vi "grabber.vi"() -> ()   [LabVIEW 2010]
uses:
  config_data_cluster.ctl
  <vilib>/Platform/TimedLoop/XDataNode/XDataNode.xnode
  <vilib>/Platform/TimedLoop/XDataNode/timing_clust.ctl
  <vilib>/Platform/TimedLoop/XDataNode/nitl_modes.ctl
  <vilib>/Platform/TimedLoop/XDataNode/wakeup.ctl
  <vilib>/dex/Flush And Wait Empty Condition.ctl
  <vilib>/rvi/interface/nirviMethod/nirviMethod.xnode
  <vilib>/rvi/interface/nirviReadWriteControl/nirviReadWriteControl.xnode
  <vilib>/rvi/interface/common/niFpgaNodeNameForErrorReporting.ctl
  <vilib>/rvi/errors/niLvFpgaWhatHappensToTopLevelVI.ctl
  <vilib>/rvi/interface/nirviCloseFPGA/nirviCloseFPGA.xnode
  <vilib>/Utility/error.llb/Error Cluster From Error Code.vi
  <vilib>/rvi/errors/niLvFpgaAdjustHostInterfaceError.vi
  <vilib>/FPGAPlugInAG/Dynamic/niLvFpga_Close_Dynamic.vi
  <vilib>/Platform/TimedLoop/XDataNode/XDNodeRunTimeDep.lvlib
  NiFpgaLv.dll
panel:
  in  "Mark fly-forward phase?":bool
  in  "adjust N sums":u32=100 max=10000 step=20
  in  "fake image fast loop?":bool
  out "ch0":u16[](graph)
  in  "Transpose graph view?":bool
  in  "Display green and red PMT?":bool
  in  "pick last TAG slice":u32
  in  "pick first TAG slice":u32
  in  "choose TAG slice?":bool
  in  "set ch1 max value":dbl
  in  "set ch0 max value":dbl
  out "ch1:position X":dbl
  out "ch0:position X":dbl
  in  "Adjust TAG phase":bool
  out "TAG profile at position X":dbl[][](graph)
  out "channel1":dbl[][](graph)
  out "channel0":dbl[][](graph)
  in  "N sums":u32(slide)=100 scale=0.0..100.0
  out "loop time":u32
  out "y galvo":i16(graph)
  out "scan specification":T1={"x amplitude"=100, "x resolution (pixels)"=28, "x offset fly-forward (iterations)"=50, "x offset fly-back (iterations)"=100, "y resolution (nr. of lines)"=80, "y step size"=30, "iterations per pixel"=5, "number of frames"=-1, "y offset (pixels)"=0, "number of y-brake lines  (before y-fly-back)"=0, "number y-brake lines (after y-fly-back)"=40, "number of y-fly-back steps"=0, "lines per z step"=1, "number of z/intensity tuples"=228, "number of repetitions (volumes or planes)"=-1, "z step size derived"=32, "choose the beginning of z scan"=FALSE, "number of frames (settings)"=80, "FPGA trajectory?"=TRUE, "Pockels cell voltage (bits)"=0, "Vy min(bits)"=0, "Vz min(bits)"=0}
  out "channel data block 2":dbl[][](graph)
  in  "fake image?":bool
  in  "xy view?":bool
  in  "Pockels cell voltage":i16(slide) min=-750 max=750 step=5 scale=-750.0..750.0
  out "DAC voltages":T2
  out "no. of extra wait lines written to FPGA FIFO":i32
  out "no. of z/int tuples written to FPGA FIFO":i32
  out "number of update commands received":i32
  out "extra wait lines set":bool
  out "zIntensity tuples set":bool
  out "scan spec set":bool
  out "display loop finished":bool
  in  "stop acquisition at FIFO overflow?  GRABBER":bool
  out "acquire?":bool
  out "FIFO overflow":bool
  out "scan":bool
  out "stop FPGA":bool
  out "wait for trigger?":bool
  out "stop acquisition at FIFO overflow?":bool
  out "scanning? FPGA":bool
  out "counter cluster out":T3
  out "extra waitlines array entries":u32[](graph)
  out "extra waitlines received by FPGA":u32
  out "no. of extra waitlines received":i32
  out "no of correctly transferred z tuples":u32
  out "z-points transfer corrupt?":bool
  out "intensity values":u16[](graph)
  out "z values":u16[](graph)
  out "no. of z/int. tubles received":i32
  out "z/intensity tuples received by FPGA":u32
  in  "wait till update":u32=500
  out "configuration":T4
  out "read FIFO overflow duration [ms]":u32
  out "read pixels duration [ms]":u32
  out "stream pixels [ms]":u32
  in  "Close front-panel?":bool=TRUE
  out "initialised?":bool
  in  "stop":bool
  out "command lp err":errorcluster
  out "error out":errorcluster
  out "effective read-block size":u32
  in  "max read block size":u32=32000
  out "read loop ctr":i32
  out "pixels read from FPGA":u64
  out "elements in FPGA FIFO":u32
  out "last received command":string
  out "command loop finished":bool
  out "read loop finished":bool
  out "scanning?":bool
  out "FIFO overflow?":bool
  out "data read from FPGA FIFO":u32[](array[numeric])
  # "enter a number between -+750V"
  # "Sum a single frame N times before displaying:"
  # "ms"
  # "automatically sets N=100 sums, otherwise FPGA buffer overflow"
  # "When T: displays and saves ch0.bin= green and ch1.bin =red\nWhen F: displays and saves ch0.bin= greenFF  and ch1.bin= greenFB  (FF=fly-forward and FB=fly-back)"
  # "Use when you want to display and save green and red PMT with marked FF and FB phases\nWhen T: fly-forward=photon counts+2^15 (number 1 at U16's most significant value)\n               and fly-back=photon counts\nWhen F: saves true photon count in both FF and FB phases of the red and green channel"
  # "How to use:\nTo adjust TAG phase\n1. set \"xy gavlo view?\"=F\n2. adjust Tag phase? = T\n3. drag cursor to desired x position\n   -- indicator below\n4. check z profile on the graph\n5. when done set N=0"
  # "How to use:\n1. set \"xy gavlo view?\"=T\n    on the main HS window\n2. to display xy view, sum all z stacks\n          set xy view?=T\n3. to choose a range of z slices to sum\na) xy view?=T\nb)choose TAG slice?=T\nc)eg. pick first Tag slice=3, pick last TAG slice=5\n   -> sums 3+4+5\nd) to display just one slice \n     set \"first=last\""
  # "RealTime Grabber"
  # "Status"
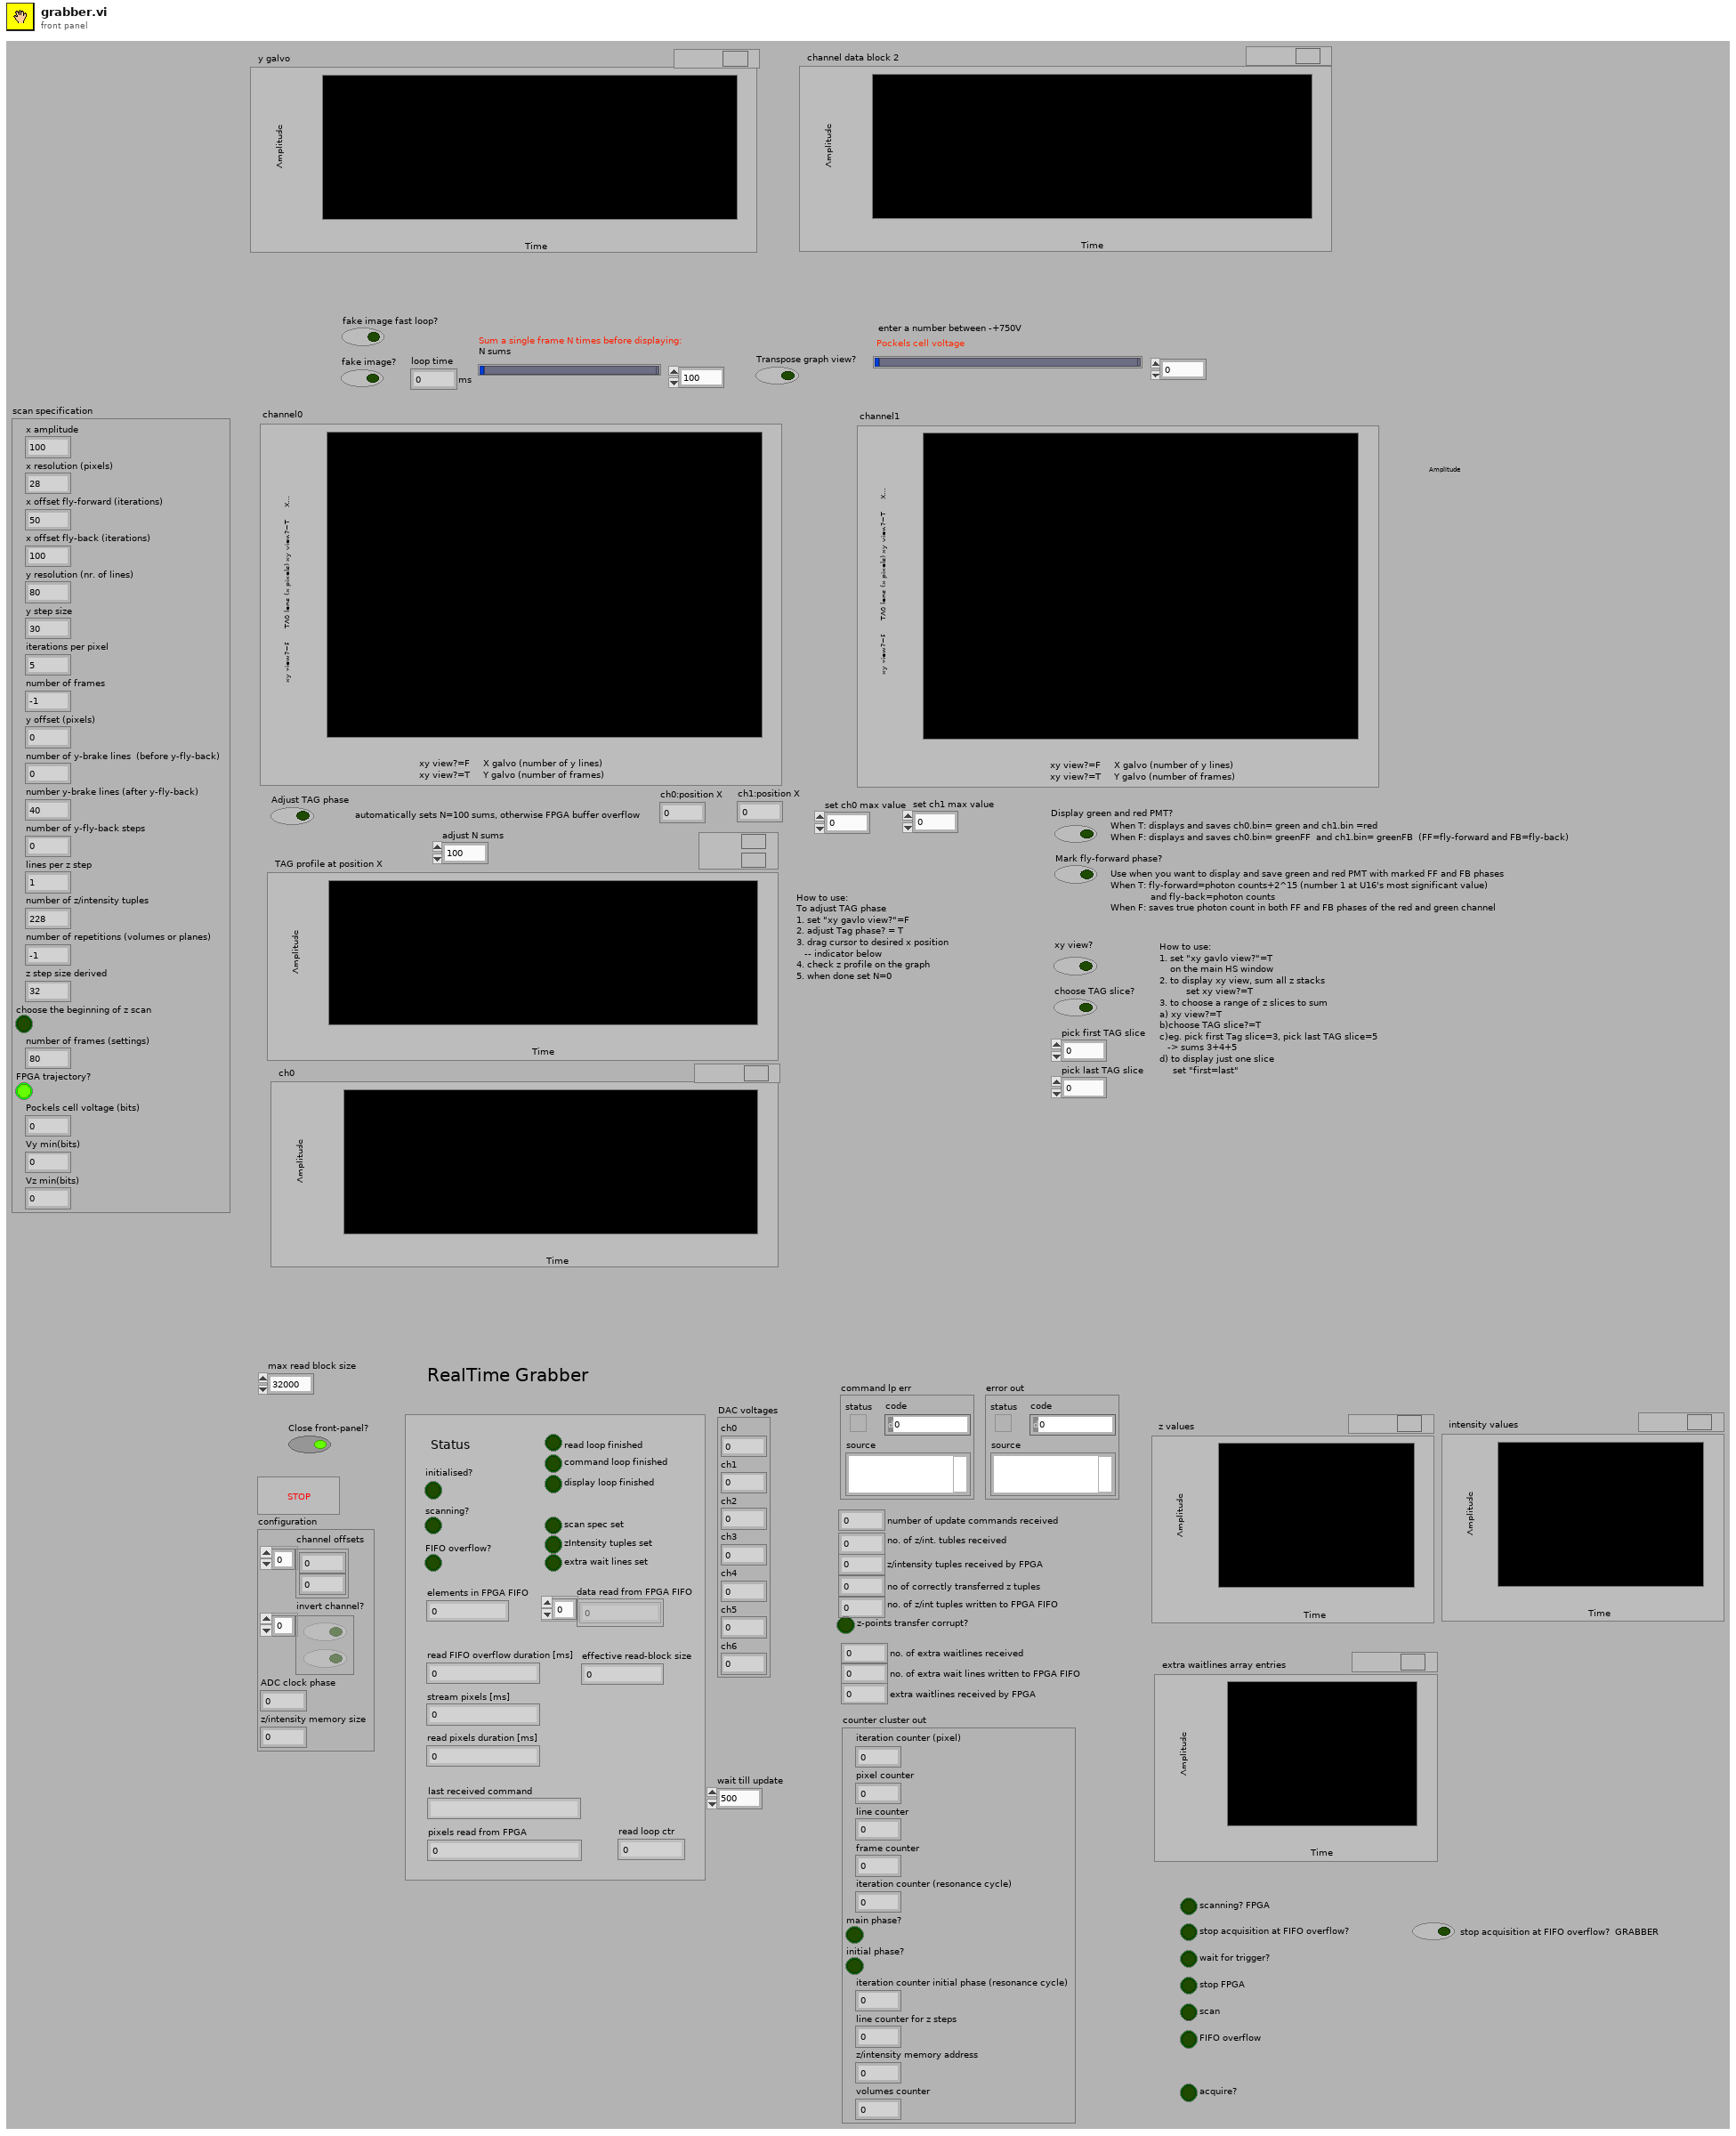
[diagram p1: front panel]
types:
  T1 = cluster{"x amplitude":u16, "x resolution (pixels)":u16, "x offset fly-forward (iterations)":u16, "x offset fly-back (iterations)":u16, "y resolution (nr. of lines)":u16, "y step size":u16, "iterations per pixel":u16, "number of frames":i32, "y offset (pixels)":u16, "number of y-brake lines  (before y-fly-back)":u16, "number y-brake lines (after y-fly-back)":u16, "number of y-fly-back steps":u16, "lines per z step":u16, "number of z/intensity tuples":u16, "number of repetitions (volumes or planes)":i32, "z step size derived":u16, "choose the beginning of z scan":bool, "number of frames (settings)":i32, "FPGA trajectory?":bool, "Pockels cell voltage (bits)":i16, "Vy min(bits)":i16, "Vz min(bits)":i16}
  T2 = cluster{"ch0":u16, "ch1":i16, "ch2":i16, "ch3":i16, "ch4":u16, "ch5":u16, "ch6":u16}
  T3 = cluster{"iteration counter (pixel)":u16, "pixel counter":u16, "line counter":u16, "frame counter":u16, "iteration counter (resonance cycle)":u16, "main phase?":bool, "initial phase?":bool, "iteration counter initial phase (resonance cycle)":u16, "line counter for z steps":u16, "z/intensity memory address":u32, "volumes counter":u16}
  T4 = typedef "config_data_cluster.ctl" = cluster{"channel offsets":u32[], "invert channel?":bool[], "ADC clock phase":i32, "z/intensity memory size":i32}
  T5 = typedef "network_streaming_queues_cluster.ctl" = cluster{"data writer endpoint":refnum<k21>, "command reader endpoint":refnum<k21>, "settings reader endpoint":refnum<k21>, "z/intensity tuples reader endpoint":refnum<k21>, "extra waitlines reader endpoint":refnum<k21>}
  T6 = typedef "XDNodeRunTimeDep.lvlib/timing_clust.ctl" = cluster{"Expected End [f-1]":u64, "Actual End [f-1]":u64, "Finished Late? [f-1]":bool, "Expected End [i-1]":u64, "Actual End [i-1]":u64, "Finished Late? [i-1]":bool, "Expected Start [i]":u64, "Actual Start [i]":u64, "Expected Start [f]":u64, "Actual Start [f]":u64, "Source Name":string, "Structure Name":string, "Period":i64, "Deadline":i64, "Offset":i64, "Start":i64, "Priority":i32, "Timeout":i32, "Mode":T7, "Wakeup Reason":T8, "Error":errorcluster, "Source Type":string, "Secondary Source Type":string, "Global End Time":u64, "Global Start Time":u64, "Frame Duration":u64, "Iteration Duration":u64, "Assigned CPU":i32, "I/O Scan Engine Mode":u32}
  T7 = typedef "XDNodeRunTimeDep.lvlib/nitl_modes.ctl" = enum32{"No Change", "Process missed periods, maintain original phase", "Discard missed periods, maintain original phase", "Process missed periods, ignore original phase", "Discard missed periods, ignore original phase"}
  T8 = typedef "XDNodeRunTimeDep.lvlib/wakeup.ctl" = enum32{"Normal", "Aborted", "Asynchronous wakeup", "Timing source error", "Timed loop error", "Timeout"}
  T9 = typedef "niFpgaNodeNameForErrorReporting.ctl" = enum16{"Open FPGA VI Reference", "Read/Write Control", "Invoke Method: Abort", "Invoke Method: Acknowledge IRQ", "Invoke Method: Download", "Invoke Method: FIFO.Configure", "Invoke Method: FIFO.Read", "Invoke Method: FIFO.Start", "Invoke Method: FIFO.Stop", "Invoke Method: FIFO.Write", "Invoke Method: Reset", "Invoke Method: Run", "Invoke Method: Wait on IRQ", "Close FPGA VI Reference"}
  T10 = typedef "niLvFpgaWhatHappensToTopLevelVI.ctl" = enum16{"top level VI scripted behind XNode", "top level VI inlined behind XNode"}
  T11 = typedef "Flush And Wait Empty Condition.ctl" = u8
  T12 = typedef "scan_specification_cluster.ctl" = cluster{"x amplitude":u16, "x resolution (pixels)":u16, "x offset fly-forward (iterations)":u16, "x offset fly-back (iterations)":u16, "y resolution (nr. of lines)":u16, "y step size":u16, "iterations per pixel":u16, "number of frames":i32, "y offset (pixels)":u16, "number of y-brake lines  (before y-fly-back)":u16, "number y-brake lines (after y-fly-back)":u16, "number of y-fly-back steps":u16, "lines per z step":u16, "number of z/intensity tuples":u16, "number of repetitions (volumes or planes)":i32, "z step size derived":u16, "choose the beginning of z scan":bool, "number of frames (settings)":i32, "FPGA trajectory?":bool, "Pockels cell voltage (bits)":i16, "Vy min(bits)":i16, "Vz min(bits)":i16}
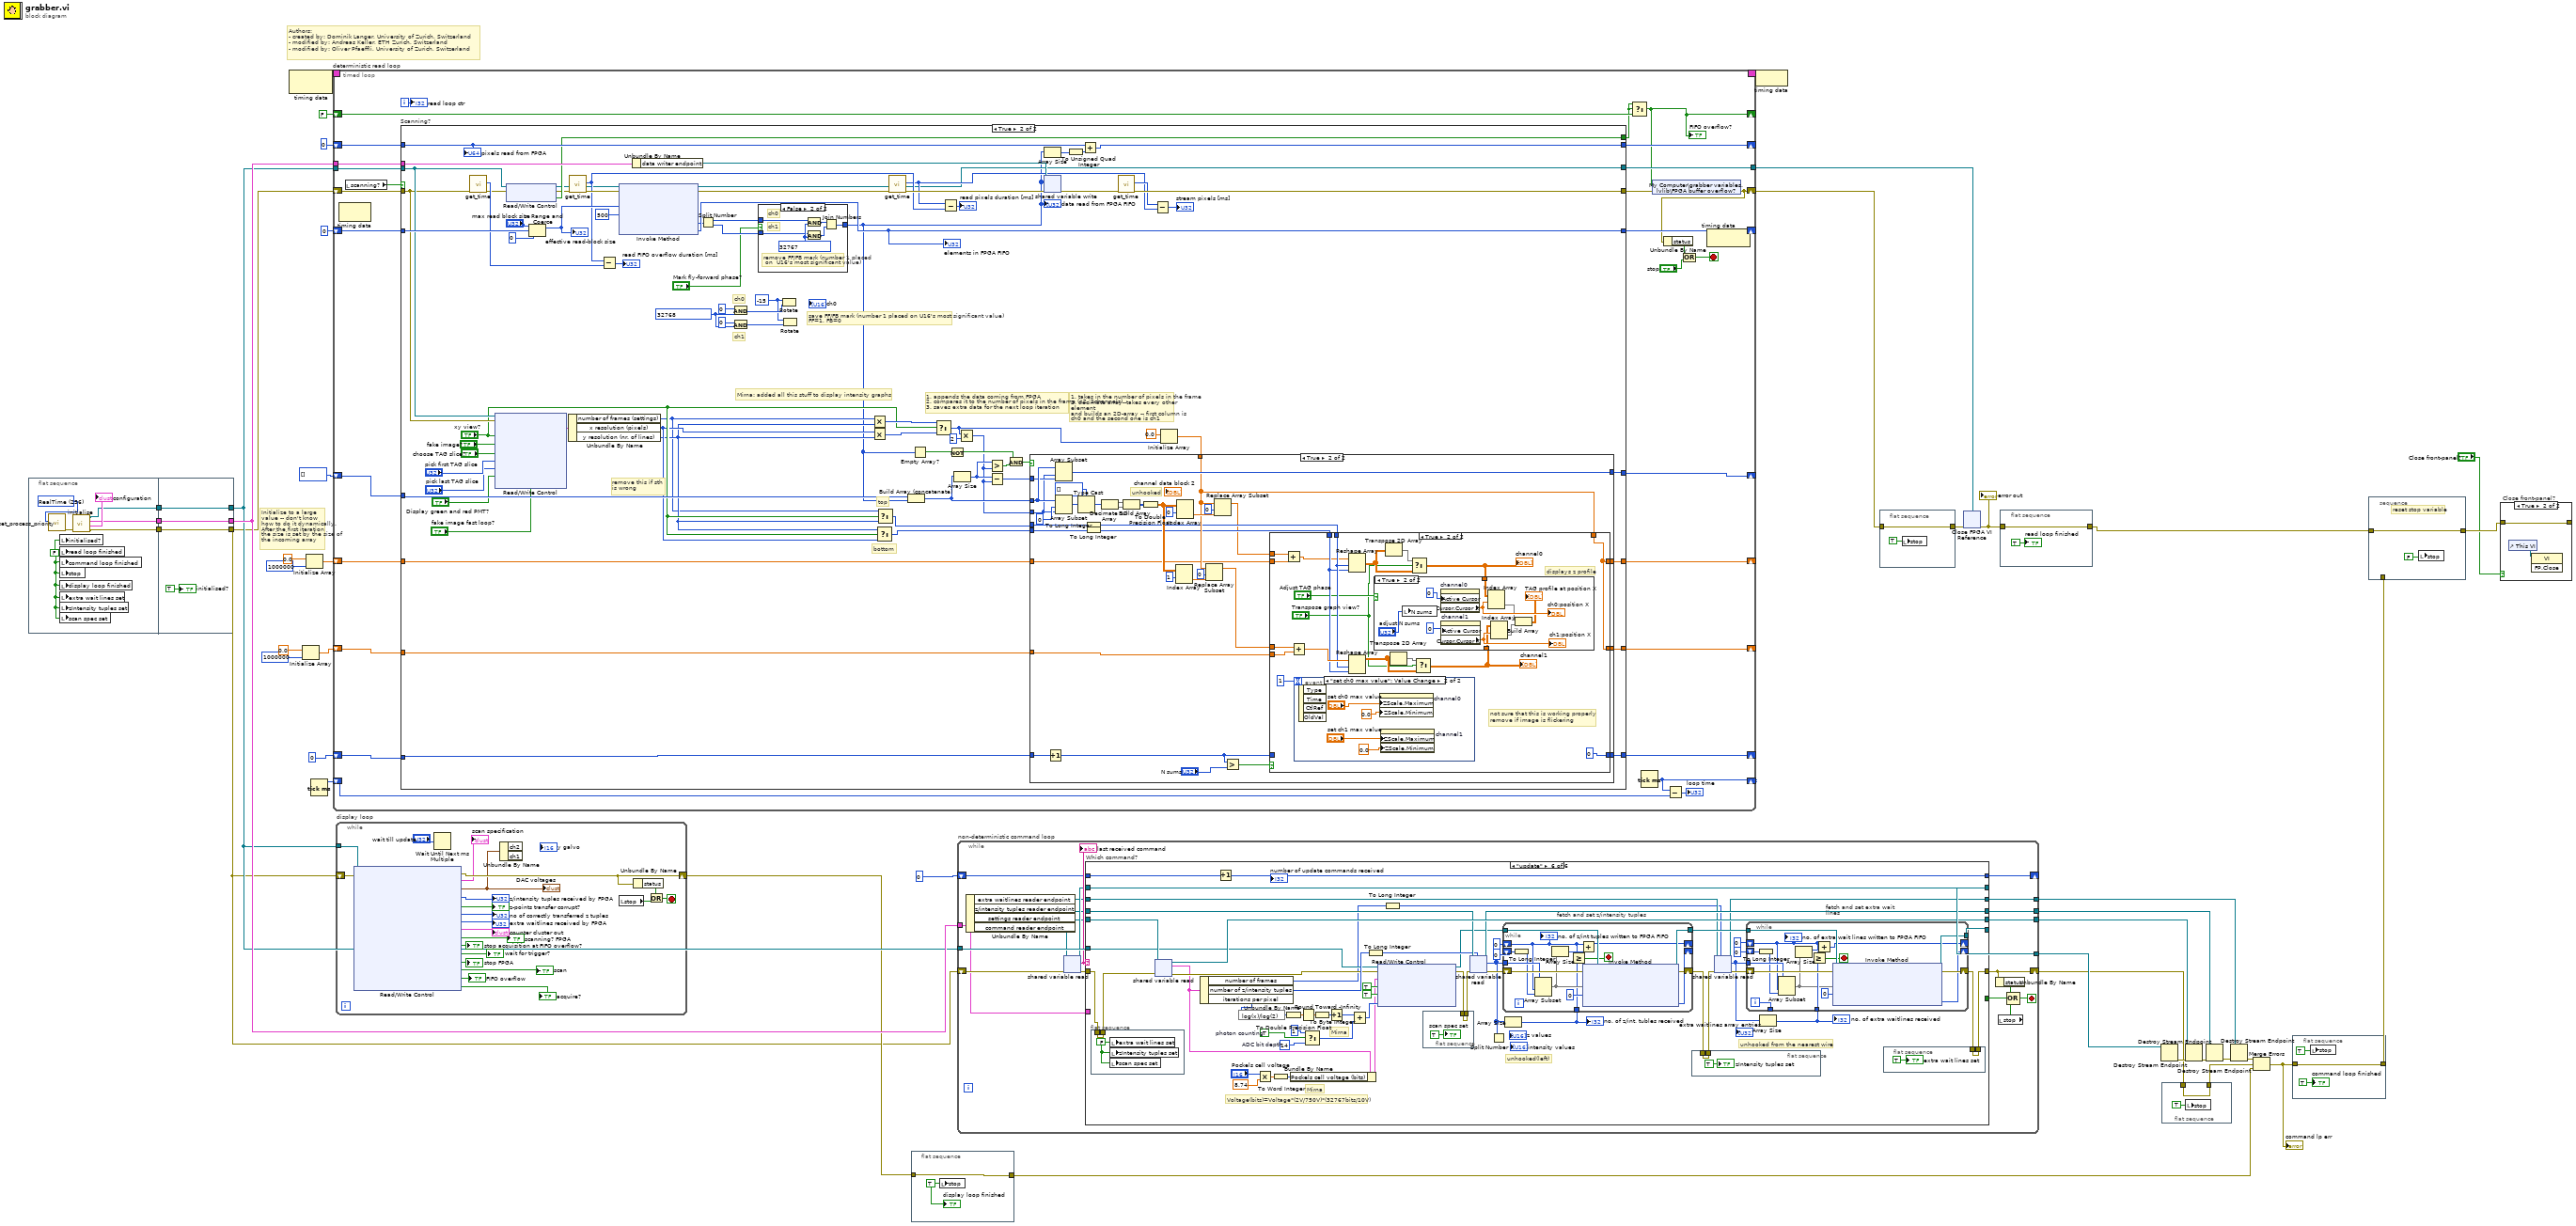
[diagram p0: block diagram]
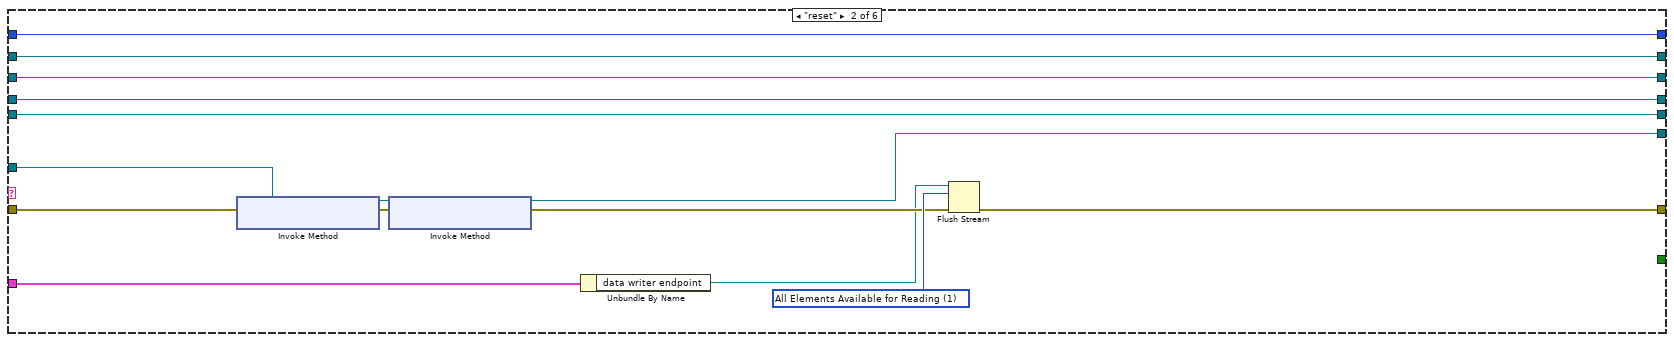
[diagram p4: hidden frame]
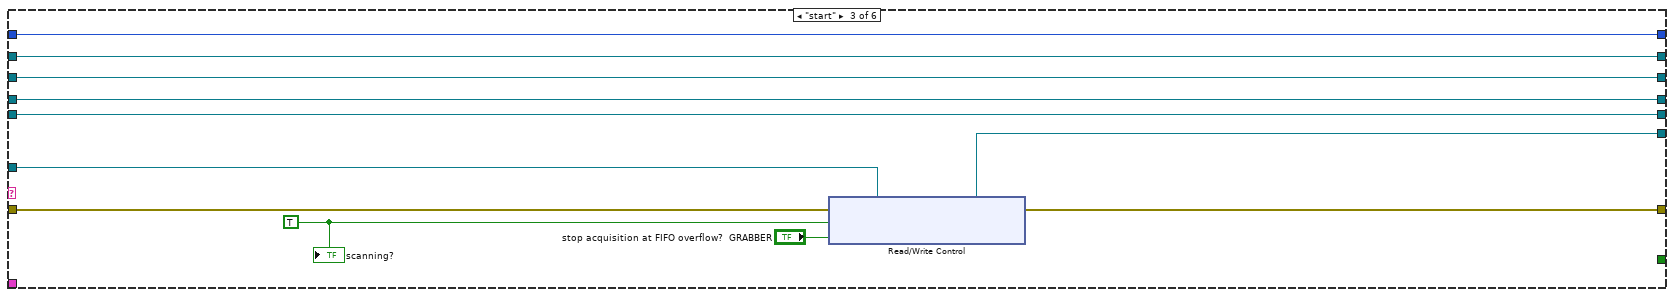
[diagram p5: hidden frame]
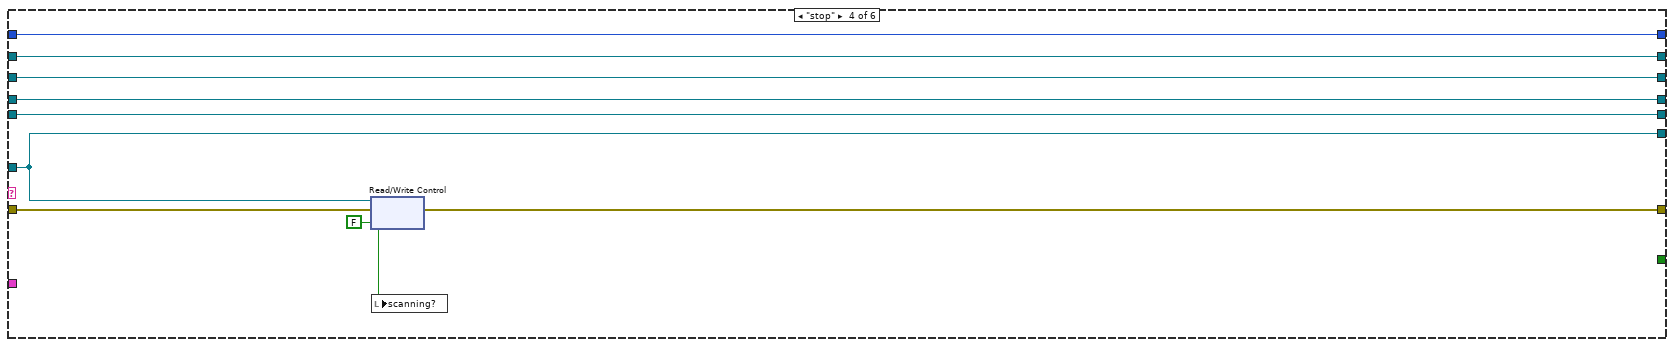
[diagram p6: hidden frame]
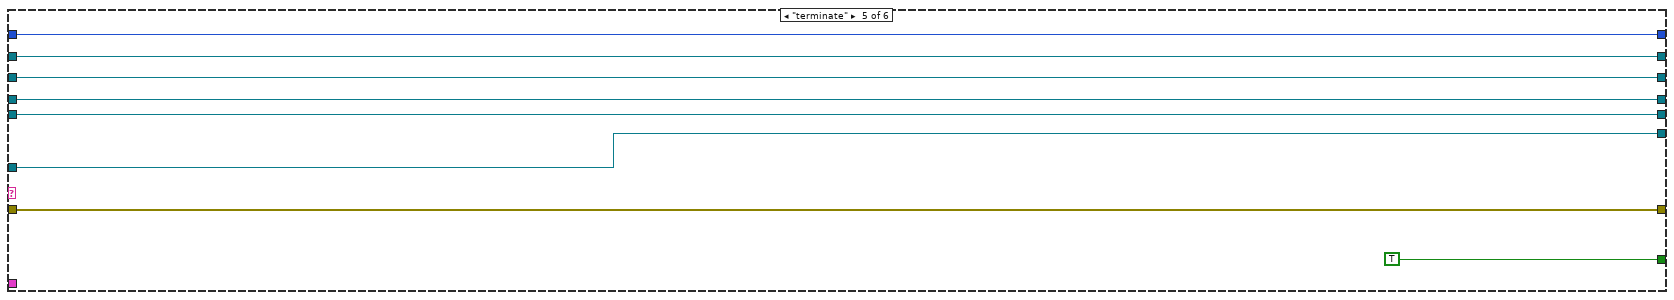
[diagram p7: hidden frame]
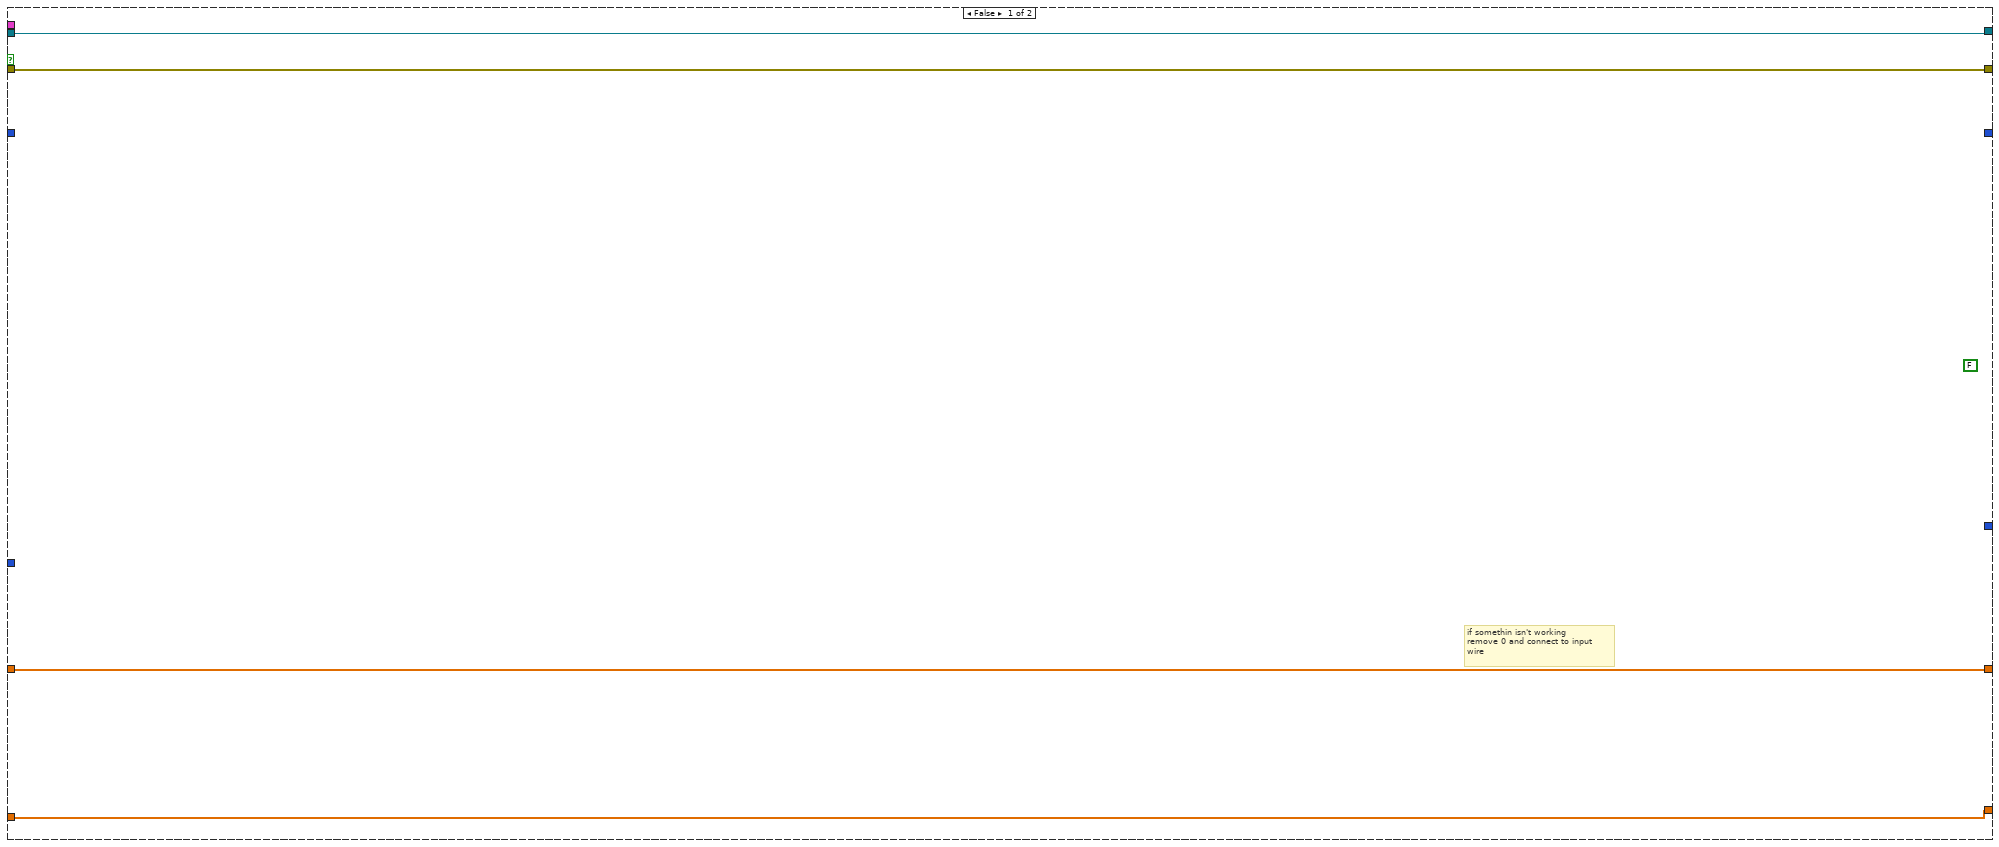
[diagram p8: hidden frame]
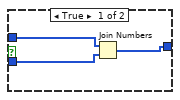
[diagram p9: hidden frame]
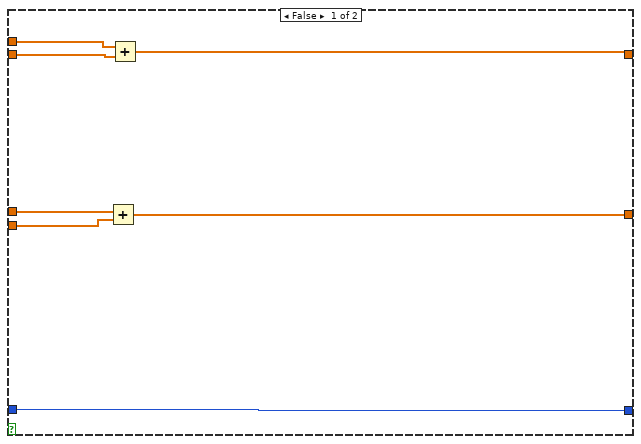
[diagram p11: hidden frame]
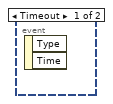
[diagram p12: hidden frame]
diagram:
  # "Initialize to a large \nvalue -- don't know \nhow to do it dynamically.\nAfter the first iteration\nthe size is set by the size of\nthe incoming array"
  # "Authors: \n- created by: Dominik Langer, University of Zurich, Switzerland\n- modified by: Andreas Keller, ETH Zurich, Switzerland\n- modified by: Oliver Pfaeffli, University of Zurich, Switzerland"
  n1 = flat-sequence {
    tunnel: [w47] -> w33
    tunnel: [w44] -> w32
    tunnel: [w45] -> w29
    tunnel: [w52] -> w22
    tunnel: [w53] -> w1
    tunnel: w33 -> [w53]
    tunnel: w32 -> [w52]
    tunnel: [w50] -> w28
    tunnel: w29 -> [w50]
    frame #0 {
      w43 = FALSE ("read loop finished")
      w49 = 256 items=["Normal"=32, "Idle"=64, "High"=128, "RealTime"=256, "BelowNormal"=16384, "AboveNormal"=32768] ("PriorityClass")
      n2 = call "set_process_priority.vi"("PriorityClass"=w49) -> ("error out"=w48:errorcluster)  [unwired: 10 in]
      n3 = local write "initialised?"(w43) -> ()
      n4 = local write "read loop finished"(w43) -> ()
      n5 = local write "command loop finished"(w43) -> ()
      n6 = local write "stop"(w43) -> ()
      n7 = local write "display loop finished"(w43) -> ()
      n8 = local write "extra wait lines set"(w43) -> ()
      n9 = local write "zIntensity tuples set"(w43) -> ()
      n10 = local write "scan spec set"(w43) -> ()
      n11 = call "initialise.vi"("error in (no error)"=w48) -> ("error out"=w47:errorcluster, "configuration"=→"configuration":T4, "network streaming queues"=w45:T5, "FPGA VI Reference Out"=w44:refnum<k20>)  [unwired: 6 in]
    }
    frame #1 {
      "initialised?" <- TRUE ("initialised?")
    }
  }
  n12 = node-c288 ("Input Node")() -> (w42:T6)  [unwired: 1 in]
  n13 = Initialize Array(0.0 ("element"), 1000000 ("dimension size")) -> (w9:dbl[])
  n14 = Initialize Array(0.0 ("element"), 1000000 ("dimension size")) -> (w3:dbl[])
  n15 = Tick Count (ms)() -> (millisecond timer value=w6:u32)
  n16 = timed-loop "deterministic read loop" {
    timing: w42 -> [_]
    timing-out: [_] -> w41
    shift-right: [w69] -> w21
    shift-left: w1 -> [w75]
    tunnel: w22 -> [w70]
    shift-right: [w56] -> _
    shift-left: FALSE ("FIFO overflow") -> [w82]
    shift-right: [w79] -> _
    shift-left: u64 0 -> [w81]
    tunnel: [w77] -> w35
    shift-right: [w73] -> _
    shift-left: u32 0 ("Elements Remaining") -> [w72]
    tunnel: w28 -> [w71]
    shift-right: [w64] -> _
    shift-left: u32[] [] -> [w65]
    shift-right: [w63] -> _
    shift-left: w9 -> [w62]
    shift-right: [w60] -> _
    shift-left: u32 0 ("Elements Remaining") -> [w61]
    shift-right: [w59] -> _
    shift-left: w6 -> [w58]
    shift-right: [w54] -> _
    shift-left: w3 -> [w55]
    i -> [w80]
    stop <- w66 stop-if-true
    n17 = node-c288 ("Output Node")() -> ()  [unwired: 1 in, 1 out]
    n18 = local read "scanning?"() -> (w74:bool)
    n19 = case "Scanning?" shown="True" w74 {
      tunnel: w75 -> [w88 w121]
      tunnel: [w88 w149] -> w76
      tunnel: w70 -> [w87 w135]
      tunnel: [w87 w137] -> w77
      tunnel: w81 -> [_ w157]
      tunnel: [_ w164] -> w79
      tunnel: [_ w140] -> w78
      tunnel: [_ w159] -> w73
      tunnel: w72 -> [_ w158]
      tunnel: w71 -> [_ w155]
      tunnel: w65 -> [_ w124]
      tunnel: [_ w123] -> w64
      tunnel: w62 -> [w85 w116]
      tunnel: [w85 w117] -> w63
      tunnel: w61 -> [_ w113]
      tunnel: [_ w115] -> w60
      tunnel: w55 -> [w86 w112]
      tunnel: [w86 w111] -> w54
      frame False {
        (unwired) FALSE ("FIFO overflow")
        # "if somethin isn't working \nremove 0 and connect to input \nwire"
      }
      frame True {
        w93 = i8 -15 ("y")
        w97 = u16 32768
        # "save FF/FB mark (number 1 placed on U16's most significant value)\nFF=1, FB=0"
        # "ch1"
        # "ch0"
        # "top"
        # "bottom"
        # "remove this if sth \nis wrong"
        # "1. takes in the number of pixels in the frame\n2. decimate array--takes every other element\nand builds an 2D-array -- first column is \nch0 and the second one is ch1"
        # "1. appends the data coming from FPGA\n2. compares it to the number of pixels in the frame (x2, 2channels)\n3. saves extra data for the next loop iteration"
        # "Mirna: added all this stuff to display intensity graphs"
        n20 = call "get_time.vi"("error in (no error)"=w121) -> ("error out"=w141:errorcluster, "millisecond timer value"=w145:u32)  [unwired: 9 in]
        n21 = xnode "Read/Write Control"("FPGA VI Reference In"=w135, "error in"=w121, "xy view?"="xy view?", "fake image?"="fake image?", "choose TAG slice?"="choose TAG slice?", "pick first TAG slice"="pick first TAG slice", "pick last TAG slice"="pick last TAG slice", "ch0-ch1?"="Display green and red PMT?", "fake image fast loop?"="fake image fast loop?") -> ("scan specification"=w136:T1)  [unwired: 2 out]
        n22 = xnode "Read/Write Control"("FPGA VI Reference In"=w135, "error in"=w141) -> ("FPGA VI Reference Out"=w138:refnum<k20>, "error out"=w139:errorcluster, "FIFO overflow"=w140:bool)
        n23 = In Range and Coerce(upper limit="max read block size", x=w158, lower limit=u32 0) -> (coerced(x)=w156:u32)  [unwired: 1 out]
        "effective read-block size" <- w156
        n24 = Unbundle By Name(w136) -> ("number of frames (settings)"=w101:i32, "x resolution (pixels)"=w104:u16, "y resolution (nr. of lines)"=w102:u16)
        n25 = call "get_time.vi"("error in (no error)"=w139) -> ("error out"=w147:errorcluster, "millisecond timer value"=w143:u32)  [unwired: 9 in]
        n26 = Subtract(x=w143, y=w145) -> (x-y=→"read FIFO overflow duration [ms]":u32)
        n27 = xnode "Invoke Method"("FPGA VI Reference In"=w138, "error in"=w147, "Number of Elements"=w156, "Timeout (ms)"=500) -> ("FPGA VI Reference Out"=w137:refnum<k20>, "error out"=w152:errorcluster, "Data"=w100:u32[], "Elements Remaining"=w159:u32)
        "elements in FPGA FIFO" <- w159
        n28 = Unbundle By Name(w155) -> ("data writer endpoint"=w154:refnum<k21>)
        n29 = Split Number(x=w100) -> (hi(x)=w98:u16[], lo(x)=w96:u16[])
        n30 = And(x=u16 0, y=w97) -> (x .and. y?=w95:u16)
        n31 = And(x=u16 0, y=w97) -> (x .and. y?=w94:u16)
        n32 = case shown="False" "Mark fly-forward phase?" {
          tunnel: [w166 w172] -> w99
          tunnel: w98 -> [w168 w170]
          tunnel: w96 -> [w167 w169]
          frame True {
            n33 = Join Numbers(hi=w168, lo=w167) -> ((hi.lo)=w166:u32[])
          }
          frame False {
            w174 = u16 32767
            # "ch1"
            # "ch0"
            # "remove FF/FB mark (number 1 placed\n on  U16's most significant value)"
            n34 = And(x=w170, y=w174) -> (x .and. y?=w173:u16[])
            n35 = And(x=w169, y=w174) -> (x .and. y?=w171:u16[])
            n36 = Join Numbers(hi=w173, lo=w171) -> ((hi.lo)=w172:u32[])
          }
        }
        "data read from FPGA FIFO" <- w99
        n37 = Rotate(1:w95, 2:w93) -> ()  [unwired: 1 out]
        n38 = Rotate(1:w94, 2:w93) -> ()  [unwired: 1 out]
        n39 = Multiply(x=w101, y=w102) -> (x*y=w119:i32)
        n40 = Multiply(x=w104, y=w102) -> (x*y=w128:u16)
        n41 = Select(t=w102, s="xy view?", f=w104) -> (s? t:f=w105:u16)
        n42 = Select(t=w101, s="xy view?", f=w102) -> (s? t:f=w103:i32)
        n43 = call "get_time.vi"("error in (no error)"=w152) -> ("error out"=w151:errorcluster, "millisecond timer value"=w142:u32)  [unwired: 9 in]
        n44 = Build Array (concatenate)(w124, w99) -> (w129:u32[])
        n45 = Empty Array?(array=w99) -> (empty?=w133:bool)
        n46 = Select(t=w119, s="xy view?", f=w128) -> (s? t:f=w120:i32)
        n47 = Subtract(x=w142, y=w143) -> (x-y=→"read pixels duration [ms]":u32)
        n48 = Not(x=w133) -> (.not. x?=w130:bool)
        n49 = Array Size(array=w129) -> (size(s)=w132:i32)
        n50 = Multiply(x=w120, y=u16 2) -> (x*y=w125:i32)
        n51 = Greater?(x=w132, y=w125) -> (0:w131:bool)
        n52 = Subtract(x=w132, y=w125) -> (x-y=w126:i32)
        n53 = And(x=w130, y=w131) -> (x .and. y?=w114:bool)
        n54 = shared-variable-write(w154, w151, w99) -> (w150:errorcluster)  [unwired: 1 in, 2 out]
        n55 = Array Size(array=w99) -> (size(s)=w165:i32)
        n56 = To Unsigned Quad Integer(1:w165) -> (0:w163:u64)
        n57 = Add(x=w157, y=w163) -> (x+y=w164:u64)
        n58 = call "get_time.vi"("error in (no error)"=w150) -> ("error out"=w149:errorcluster, "millisecond timer value"=w148:u32)  [unwired: 9 in]
        n59 = Subtract(x=w148, y=w142) -> (x-y=→"stream pixels [ms]":u32)
        n60 = Initialize Array(0.0 ("element"), w120) -> (w118:dbl[])
        n61 = case shown="True" w114 {
          tunnel: w129 -> [w178 w211]
          tunnel: w125 -> [_ w209]
          tunnel: w126 -> [_ w210]
          tunnel: [w178 w208] -> w123
          tunnel: w103 -> [_ w202]
          tunnel: w105 -> [_ w201]
          tunnel: w118 -> [_ w187]
          tunnel: w116 -> [w177 w194]
          tunnel: [w177 w189] -> w117
          tunnel: [w176 w193] -> w115
          tunnel: w113 -> [w176 w192]
          tunnel: w112 -> [w175 w181]
          tunnel: [w175 w180] -> w111
          frame False {
          }
          frame True {
            # "unhooked"
            n62 = Increment(x=w192) -> (x+1=w179:u32)
            n63 = Array Subset(array=w211, index=w209, length=w210) -> (w208:u32[])
            n64 = Array Subset(array=w211, index=0, length=w209) -> (w196:u32[])
            n65 = Type Cast(type=u16[] [], x=w196) -> (*(type *) &x=w205:u16[])
            n66 = To Long Integer(number=w202) -> (32bit integer=w186:i32)
            n67 = To Long Integer(number=w201) -> (32bit integer=w185:i32)
            n68 = Decimate 1D Array(w205) -> (w207:u16[], w206:u16[])
            n69 = Build Array(w207, w206) -> (w204:u16[][])
            n70 = To Double Precision Float(number=w204) -> (double precision float=w200:dbl[][])
            n71 = Index Array(array=w200, index (row)=1 ("index (col)")) -> (element=w190:dbl[])  [unwired: 1 in]
            n72 = Index Array(array=w200, index (row)=0) -> (element=w198:dbl[])  [unwired: 1 in]
            n73 = Replace Array Subset(array=w187, new element=w190, index=0) -> (w183:dbl[])
            n74 = Replace Array Subset(array=w187, new element=w198, index=0) -> (w182:dbl[])
            n75 = Greater?(x=w179, y="N sums") -> (0:w188:bool)
            n76 = case shown="True" w188 {
              tunnel: w194 -> [w216 w238]
              tunnel: [w219 u32 0] -> w193
              tunnel: w183 -> [w218 w237]
              tunnel: [w217 w230] -> w189
              tunnel: w179 -> [w219 _]
              tunnel: w187 -> [_ w230]
              tunnel: w186 -> [_ w234]
              tunnel: w185 -> [_ w233]
              tunnel: w182 -> [w215 w232]
              tunnel: w181 -> [w214 w231]
              tunnel: [w213 w230] -> w180
              frame False {
                n77 = Add(x=w218, y=w216) -> (x+y=w217:dbl[])
                n78 = Add(x=w215, y=w214) -> (x+y=w213:dbl[])
              }
              frame True {
                # "displays z profile"
                # "not sure that this is working properly\nremove if image is flickering"
                n79 = Add(x=w232, y=w231) -> (x+y=w228:dbl[])
                n80 = Add(x=w237, y=w238) -> (x+y=w235:dbl[])
                n81 = event shown="[1] \"set ch0 max value\": Value Change" {
                  selector: _ -> [_ _]
                  dyn-events: _ -> [_ _]
                  timeout: 1 -> [_ _]
                  event Timeout {
                    n82 = event-data() -> ()  [unwired: 1 in, 2 out]
                  }
                  event "set ch0 max value": Value Change {
                    n83 = event-data() -> ()  [unwired: 1 in, 4 out]
                    n84 = property on="channel0" class="IntGraph (strict)"("ZScale.Maximum"="set ch0 max value", "ZScale.Minimum"=0.0 ("Z Scale.Range:Minimum")) -> ()  [unwired: 2 in, 2 out]
                    n85 = property on="channel1" class="IntGraph (strict)"("ZScale.Maximum"="set ch1 max value", "ZScale.Minimum"=0.0 ("Z Scale.Range:Minimum")) -> ()  [unwired: 2 in, 2 out]
                  }
                }
                n86 = Reshape Array(w228, w234, w233) -> (w224:dbl[][])
                n87 = Reshape Array(w235, w234, w233) -> (w221:dbl[][])
                n88 = Transpose 2D Array(2D array=w224) -> (transposed array=w226:dbl[][])
                n89 = Transpose 2D Array(2D array=w221) -> (transposed array=w223:dbl[][])
                n90 = Select(t=w226, s="Transpose graph view?", f=w224) -> (s? t:f=w225:dbl[][])
                "channel0" <- w225
                n91 = Select(t=w223, s="Transpose graph view?", f=w221) -> (s? t:f=w222:dbl[][])
                "channel1" <- w222
                n92 = case shown="True" "Adjust TAG phase" {
                  tunnel: w225 -> [_ w251]
                  tunnel: w222 -> [_ w245]
                  frame False {
                  }
                  frame True {
                    n93 = local write "N sums"("adjust N sums") -> ()
                    n94 = property on="channel0" class="IntGraph (strict)"("Active Cursor"=u32 0) -> ("Cursor.Cursor X"=w250:dbl)  [unwired: 2 in, 2 out]
                    "ch0:position X" <- w250
                    n95 = property on="channel1" class="IntGraph (strict)"("Active Cursor"=u32 0) -> ("Cursor.Cursor X"=w248:dbl)  [unwired: 2 in, 2 out]
                    "ch1:position X" <- w248
                    n96 = Index Array(array=w251, index (row)=w250) -> (element=w247:dbl[])  [unwired: 1 in]
                    n97 = Index Array(array=w245, index (row)=w248) -> (element=w246:dbl[])  [unwired: 1 in]
                    n98 = Build Array(w247, w246) -> (→"TAG profile at position X":dbl[][])
                  }
                }
              }
            }
          }
        }
        "pixels read from FPGA" <- w157
      }
    }
    n99 = Select(t=w78, s=w78, f=w82) -> (s? t:f=w56:bool)
    "FIFO overflow?" <- w56
    n100 = Tick Count (ms)() -> (millisecond timer value=w59:u32)
    n101 = shared-variable "My Computer\\grabber variables.lvlib\\FPGA buffer overflow?"(w56, error in=w76) -> (error out=w69:errorcluster)
    n102 = Unbundle By Name(w69) -> ("status"=w68:bool)
    n103 = Subtract(x=w59, y=w58) -> (x-y=→"loop time":u32)
    n104 = Compound Arithmetic op=OR(w68, "stop") -> (w66:bool)
    n105 = node-c288 ("Input Node")() -> ()  [unwired: 1 in, 1 out]
    "read loop ctr" <- w80
  }
  n106 = while "display loop" {
    tunnel: w22 -> [w591]
    shift-right: [w589] -> w19
    shift-left: w1 -> [w590]
    stop <- w586 stop-if-true
    n107 = xnode "Read/Write Control"("FPGA VI Reference In"=w591, "error in"=w590) -> ("error out"=w589:errorcluster, "scan specification"=→"scan specification":T1, "DAC voltages"=w572:T2, "transferred z/intensity tuples"=→"z/intensity tuples received by FPGA":u32, "z-points transfer corrupt?"=→"z-points transfer corrupt?":bool, "no of correct transferred z tuples"=→"no of correctly transferred z tuples":u32, "transferred extra waitlines"=→"extra waitlines received by FPGA":u32, "counter cluster out"=→"counter cluster out":T3, "scanning?"=→"scanning? FPGA":bool, "stop acquisition at FIFO overflow?"=→"stop acquisition at FIFO overflow?":bool, "wait for trigger?"=→"wait for trigger?":bool, "stop"=→"stop FPGA":bool, "scan"=→"scan":bool, "FIFO overflow"=→"FIFO overflow":bool, "acquire?"=→"acquire?":bool)  [unwired: 1 out]
    "DAC voltages" <- w572
    n108 = Wait Until Next ms Multiple(millisecond multiple="wait till update") -> ()  [unwired: 1 out]
    n109 = Unbundle By Name(w572) -> ()  [unwired: 2 out]
    n110 = local read "stop"() -> (w587:bool)
    n111 = Unbundle By Name(w589) -> ("status"=w588:bool)
    n112 = Or(x=w588, y=w587) -> (x .or. y?=w586:bool)
  }
  n113 = flat-sequence {
    tunnel: w19 -> [w983]
    tunnel: [w983] -> w18
    frame #0 {
      w982 = TRUE ("stop")
      n114 = local write "stop"(w982) -> ()
      "display loop finished" <- w982
    }
  }
  n115 = while "non-deterministic command loop" {
    shift-right: [w991] -> w17
    shift-left: w1 -> [w1004]
    tunnel: w22 -> [w1003]
    tunnel: [w999] -> w40
    tunnel: w28 -> [w997]
    tunnel: [w995] -> w25
    tunnel: [w993] -> w23
    tunnel: [w986] -> w13
    shift-right: [w984] -> _
    shift-left: 0 -> [w985]
    stop <- w989 stop-if-true
    n116 = Unbundle By Name(w997) -> ("extra waitlines reader endpoint"=w987:refnum<k21>, "z/intensity tuples reader endpoint"=w994:refnum<k21>, "settings reader endpoint"=w996:refnum<k21>, "command reader endpoint"=w998:refnum<k21>)
    n117 = shared-variable-read(w998, w1004) -> (w1000:refnum<k21>, w1002:errorcluster, w1001:string)  [unwired: 1 in, 1 out]
    "last received command" <- w1001
    n118 = case "Which command?" shown="\"update\"" w1001 {
      tunnel: w1003 -> [w1009 w1024 w1079 w1150 w1197 w1238]
      tunnel: w1002 -> [w1011 w1026 w1077 w1149 w1196 w1215]
      tunnel: [w1011 w1018 w1081 w1147 w1196 w1220] -> w991
      tunnel: w1000 -> [w1010 w1025 w1080 w1151 w1198 w1248]
      tunnel: [w1010 w1025 w1080 w1151 w1198 w1248] -> w999
      tunnel: [w1009 w1023 w1078 w1150 w1197 w1229] -> _
      tunnel: w997 -> [_ w1017 _ _ _ _]
      tunnel: w996 -> [w1008 w1015 w1075 w1146 w1195 w1247]
      tunnel: [w1008 w1015 w1075 w1146 w1195 w1246] -> w995
      tunnel: w994 -> [w1007 w1014 w1074 w1145 w1194 w1245]
      tunnel: [w1007 w1014 w1074 w1145 w1194 w1244] -> w993
      tunnel: [_ _ _ _ TRUE _] -> w992
      tunnel: w987 -> [w1006 w1013 w1073 w1144 w1192 w1227]
      tunnel: [w1006 w1013 w1073 w1144 w1192 w1226] -> w986
      tunnel: w985 -> [w1005 w1012 w1071 w1143 w1191 w1213]
      tunnel: [w1005 w1012 w1071 w1143 w1191 w1212] -> w984
      frame "NULL", Default {
      }
      frame "reset" {
        w1020 = T11 1 items=["All Elements Read From Stream", "All Elements Available for Reading"] ("wait condition")
        n119 = xnode "Invoke Method"("FPGA VI Reference In"=w1024, "error in"=w1026) -> ("FPGA VI Reference Out"=w1021:refnum<k20>, "error out"=w1022:errorcluster)
        n120 = xnode "Invoke Method"("FPGA VI Reference In"=w1021, "error in"=w1022) -> ("FPGA VI Reference Out"=w1023:refnum<k20>, "error out"=w1019:errorcluster)
        n121 = Unbundle By Name(w1017) -> ("data writer endpoint"=w1016:refnum<k21>)
        n122 = Flush Stream(8:w1019, 10:w1020, 11:w1016) -> (0:w1018:errorcluster)  [unwired: 1 in, 2 out]
      }
      frame "start" {
        w1076 = TRUE ("scan")
        n123 = xnode "Read/Write Control"("FPGA VI Reference In"=w1079, "error in"=w1077, "scan"=w1076, "stop acquisition at FIFO overflow?"="stop acquisition at FIFO overflow?  GRABBER") -> ("FPGA VI Reference Out"=w1078:refnum<k20>, "error out"=w1081:errorcluster)
        "scanning?" <- w1076
      }
      frame "stop" {
        w1148 = FALSE ("scan")
        n124 = xnode "Read/Write Control"("FPGA VI Reference In"=w1150, "error in"=w1149, "scan"=w1148) -> ("error out"=w1147:errorcluster)  [unwired: 1 out]
        n125 = local write "scanning?"(w1148) -> ()
      }
      frame "terminate" {
      }
      frame "update" {
        w1207 = TRUE  # photon counting
        w1211 = i8 14  # ADC bit depth
        # "unhooked from the nearest wire"
        # "unhooked(left)"
        # "Mirna"
        # "Voltage(bits)=Voltage*(2V/750V)*(32767bits/10V)"
        # "Mirna"
        n126 = flat-sequence {
          tunnel: w1215 -> [w1254]
          tunnel: [w1254] -> w1214
          frame #0 {
            w1255 = FALSE ("extra wait lines set")
            n127 = local write "extra wait lines set"(w1255) -> ()
            n128 = local write "zIntensity tuples set"(w1255) -> ()
            n129 = local write "scan spec set"(w1255) -> ()
          }
        }
        n130 = shared-variable-read(w1247, w1214) -> (w1246:refnum<k21>, w1240:errorcluster, w1202:T12)  [unwired: 1 in, 1 out]
        n131 = Unbundle By Name(w1202) -> ("number of frames"=w1225:i32, "number of z/intensity tuples"=w1243:u16, "iterations per pixel"=w1201:u16)
        n132 = Increment(x=w1213) -> (x+1=w1212:i32)
        "number of update commands received" <- w1212
        n133 = expression code="log(x)/log(2)"(w1201) -> (w1249:u16)
        n134 = Multiply(x="Pockels cell voltage", y=8.74 ("x")) -> (x*y=w1204:dbl)
        n135 = To Word Integer(number=w1204) -> (16bit integer=w1203:i16)
        n136 = To Double Precision Float(number=w1249) -> (double precision float=w1251:dbl)
        n137 = Bundle By Name(cluster=w1202, "Pockels cell voltage (bits)"=w1203) -> (w1200:T12)
        n138 = Round Toward -Infinity(1:w1251) -> (0:w1250:dbl)
        n139 = Select(t=i8 1, s=w1207, f=w1211) -> (s? t:f=w1209:i8)
        n140 = To Byte Integer(number=w1250) -> (8bit integer=w1252:i8)
        n141 = Increment(x=w1252) -> (x+1=w1253:i8)
        n142 = Add(x=w1253, y=w1209) -> (x+y=w1233:i8)
        n143 = To Long Integer(number=w1243) -> (32bit integer=w1242:i32)
        n144 = xnode "Read/Write Control"("FPGA VI Reference In"=w1238, "error in"=w1240, "scan specification"=w1200, "transfer z-points?"=TRUE, "transfer extra-waitlines?"=TRUE ("transfer z-points?"), "maximum bit depth"=w1233) -> ("FPGA VI Reference Out"=w1239:refnum<k20>, "error out"=w1217:errorcluster)
        n145 = To Long Integer(number=w1225) -> (32bit integer=w1224:i32)
        n146 = flat-sequence {
          tunnel: [w1260] -> w1216
          tunnel: w1217 -> [w1260]
          frame #0 {
            "scan spec set" <- TRUE ("zIntensity tuples set")
          }
        }
        n147 = shared-variable-read(w1245, w1216, w1242) -> (w1244:refnum<k21>, w1241:errorcluster, w1237:u32[])  [unwired: 1 in, 1 out]
        n148 = Split Number(x=w1237) -> ()  [unwired: 2 out]
        n149 = Array Size(array=w1237) -> (size(s)=w1236:i32)
        "no. of z/int. tubles received" <- w1236
        n150 = while "fetch and set z/intensity tuples" {
          tunnel: [w1357] -> w1230
          tunnel: w1239 -> [w1356]
          shift-right: [w1354] -> _
          shift-left: u32 0 ("Empty Elements Remaining") -> [w1352]
          tunnel: w1237 -> [w1353]
          shift-right: [w1350] -> _
          shift-left: 0 -> [w1347]
          tunnel: w1236 -> [w1346]
          shift-right: [w1358] -> w1219
          shift-left: w1241 -> [w1359]
          stop <- w1345 stop-if-true
          n151 = To Long Integer(number=w1352) -> (32bit integer=w1351:i32)
          n152 = Array Subset(array=w1353, index=w1347, length=w1351) -> (w1348:u32[])
          n153 = Array Size(array=w1348) -> (size(s)=w1349:i32)
          n154 = Greater Or Equal?(x=w1347, y=w1346) -> (x >= y?=w1345:bool)
          n155 = Add(x=w1347, y=w1349) -> (x+y=w1350:i32)
          n156 = xnode "Invoke Method"("FPGA VI Reference In"=w1356, "error in"=w1359, "Data"=w1348, "Timeout (ms)"=0) -> ("FPGA VI Reference Out"=w1357:refnum<k20>, "error out"=w1358:errorcluster, "Empty Elements Remaining"=w1354:u32)
          "no. of z/int tuples written to FPGA FIFO" <- w1347
        }
        n157 = flat-sequence {
          tunnel: [w1258] -> w1218
          tunnel: w1219 -> [w1258]
          frame #0 {
            "zIntensity tuples set" <- TRUE ("scan spec set")
          }
        }
        n158 = shared-variable-read(w1227, w1218, w1224) -> (w1226:refnum<k21>, w1228:errorcluster, w1199:u32[])  [unwired: 1 in, 1 out]
        n159 = Array Size(array=w1199) -> (size(s)=w1223:i32)
        "no. of extra waitlines received" <- w1223
        n160 = while "fetch and set extra wait lines" {
          shift-right: [w1266] -> _
          shift-left: 0 -> [w1263]
          shift-right: [w1267] -> _
          shift-left: u32 0 ("Empty Elements Remaining") -> [w1272]
          tunnel: w1230 -> [w1277]
          tunnel: [w1276] -> w1229
          tunnel: w1199 -> [w1273]
          tunnel: w1223 -> [w1269]
          shift-right: [w1274] -> w1221
          shift-left: w1228 -> [w1275]
          tunnel: [w1262] -> _
          i -> [w1262]
          stop <- w1268 stop-if-true
          n161 = To Long Integer(number=w1272) -> (32bit integer=w1271:i32)
          n162 = Array Subset(array=w1273, index=w1263, length=w1271) -> (w1265:u32[])
          n163 = Array Size(array=w1265) -> (size(s)=w1270:i32)
          n164 = Greater Or Equal?(x=w1263, y=w1269) -> (x >= y?=w1268:bool)
          n165 = Add(x=w1263, y=w1270) -> (x+y=w1266:i32)
          n166 = xnode "Invoke Method"("FPGA VI Reference In"=w1277, "error in"=w1275, "Data"=w1265, "Timeout (ms)"=0) -> ("FPGA VI Reference Out"=w1276:refnum<k20>, "error out"=w1274:errorcluster, "Empty Elements Remaining"=w1267:u32)
          "no. of extra wait lines written to FPGA FIFO" <- w1263
        }
        n167 = flat-sequence {
          tunnel: w1221 -> [w1256]
          tunnel: [w1256] -> w1220
          frame #0 {
            "extra wait lines set" <- TRUE ("extra wait lines set")
          }
        }
      }
    }
    n168 = Unbundle By Name(w991) -> ("status"=w990:bool)
    n169 = local read "stop"() -> (w988:bool)
    n170 = Compound Arithmetic op=OR(w990, w992, w988) -> (w989:bool)
  }
  n171 = node-c288 ("Output Node")(w41) -> ()
  n172 = flat-sequence {
    tunnel: w21 -> [w1536]
    tunnel: [w1536] -> w20
    frame #0 {
      n173 = local write "stop"(TRUE ("stop")) -> ()
    }
  }
  n174 = xnode "Close FPGA VI Reference"("FPGA VI Reference In"=w35, "error in"=w20) -> ("error out"=w27:errorcluster)
  "error out" <- w27
  n175 = flat-sequence {
    tunnel: w27 -> [w1539]
    tunnel: [w1539] -> w38
    frame #0 {
      "read loop finished" <- TRUE ("read loop finished")
    }
  }
  n176 = Destroy Stream Endpoint(11:w40) -> (0:w26:errorcluster)  [unwired: 1 in]
  n177 = flat-sequence {
    tunnel: [w1540] -> w16
    tunnel: w17 -> [w1540]
    frame #0 {
      n178 = local write "stop"(TRUE ("stop")) -> ()
    }
  }
  n179 = Destroy Stream Endpoint(8:w26, 11:w25) -> (0:w24:errorcluster)
  n180 = Destroy Stream Endpoint(8:w24, 11:w23) -> (0:w15:errorcluster)
  n181 = Destroy Stream Endpoint(8:w15, 11:w13) -> (0:w14:errorcluster)
  n182 = Merge Errors(w14, w16, w18) -> (w34:errorcluster)
  "command lp err" <- w34
  n183 = flat-sequence {
    tunnel: w34 -> [w1542]
    tunnel: [w1542] -> w39
    frame #0 {
      n184 = local write "stop"(TRUE ("stop - RT")) -> ()
      "command loop finished" <- TRUE ("command loop finished")
    }
  }
  n185 = stacked-sequence {
    tunnel: w39 -> [_]
    tunnel: w38 -> [w1545]
    tunnel: [w1545] -> w31
    frame #0 {
      # "reset stop variable"
      n186 = local write "stop"(FALSE) -> ()
    }
  }
  n187 = case "Close front-panel?" shown="True" "Close front-panel?" {
    tunnel: [w1547 w1548] -> _
    tunnel: w31 -> [w1547 w1548]
    frame False {
    }
    frame True {
      n188 = control-ref of="This VI"() -> (w1549:refnum<vi>)
      n189 = invoke class="VI" method="FP.Close"(reference=w1549) -> ()  [unwired: 2 in, 3 out]
    }
  }
